vi "distancepidinit.vi"(10 "Distance From Target":dbl) -> (1 "Done?":bool)   [LabVIEW 2013]
uses:
  <vilib>/addons/control/pid/pid.llb/PID (DBL).vi
  <vilib>/Rock Robotics/WPI/RobotDrive/WPI_RobotDriveArcadeDrive_Standard(NoSaturation).vi
  <vilib>/Rock Robotics/WPI/RobotDrive/WPI_RobotDriveGetSetRefNum.vi
  <vilib>/addons/control/pid/NI_PID_pid.lvlib
panel:
  in  "reinitialize? (F)":bool
  in  "PID Gains Distance":T1={"proportional gain (Kc)"=0.3, "integral time (Ti, min)"=0.0, "derivative time (Td, min)"=0.0} {"derivative time (Td, min)" format="%.3f"; "integral time (Ti, min)" format="%.3f"; "proportional gain (Kc)" format="%.3f"}
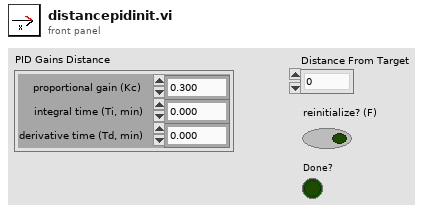
[diagram p1: front panel]
types:
  T1 = cluster{"proportional gain (Kc)":dbl, "integral time (Ti, min)":dbl, "derivative time (Td, min)":dbl}
  T2 = typedef "WPI_EncoderDevRef.ctl" = cluster{"DevStatus":errorcluster, "EncoderIndex":T3, "CounterIndex":T4, "DistancePerCount":dbl, "Decoding Type":T5}
  T3 = typedef "FPGA_EncoderIdx.ctl" = enum8{"Enc 0", "Enc 1", "Enc 2", "Enc 3", "Invalid"}
  T4 = typedef "FPGA_CounterCtrSystemIndex.ctl" = enum8{"Ctr 0", "Ctr 1", "Ctr 2", "Ctr 3", "Ctr 4", "Ctr 5", "Ctr 6", "Ctr 7", "Invalid"}
  T5 = typedef "WPI_EncoderType.ctl" = enum16{"1x", "2x", "4x"}
  T6 = typedef "WPI_RobotDriveDevRef.ctl" = cluster{"DevStatus":errorcluster, "Motors[]":T7[], "Square Inputs":bool, "Max Output":dbl, "Isochronous":bool}
  T7 = typedef "WPI_MotorControlDeviceRef.ctl" = cluster{"DeviceStatus":errorcluster, "Type":enum16{"PWM", "CAN"}, "PWM":cluster{"Digital Module":T8, "PWM Channel":T9, "DeadBand":T10}, "CAN":cluster{"Device Number":u8, "Control Mode":T11, "Semaphore":T12, "Max Vout":dbl}, "Invert":bool, "TransformRef":T13, "InvTransformRef":T13}
  T8 = typedef "FPGA_TypedefDigitalModule.ctl" = enum16{"Digital Module 1", "Digital Module 2"}
  T9 = typedef "FPGA_DIOPWMChannel.ctl" = enum8{"PWM 1", "PWM 2", "PWM 3", "PWM 4", "PWM 5", "PWM 6", "PWM 7", "PWM 8", "PWM 9", "PWM 10", "Invalid"}
  T10 = typedef "WPI_PWMDeadband.ctl" = cluster{"Name":string, "maxPositivePwm":i32, "minPositivePwm":i32, "centerPwm":i32, "maxNegativePwm":i32, "minNegativePwm":i32, "angularRange":u16}
  T11 = typedef "WPI_CANJaguar_ControlMode.ctl" = enum8{"Percent VBus", "Current", "Speed", "Position", "Voltage"}
  T12 = typedef "Semaphore RefNum" = refnum<k1>
  T13 = typedef "WPI_PWMTransform_ConPane.ctl" = refnum<vi>
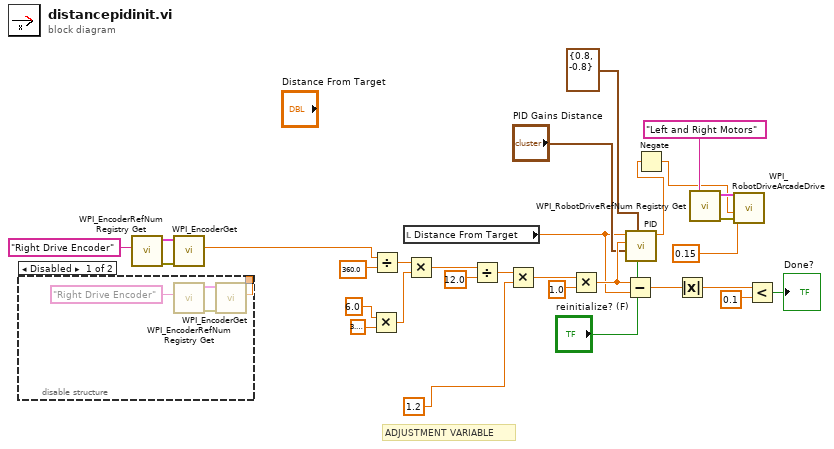
[diagram p0: block diagram]
diagram:
  # "ADJUSTMENT VARIABLE"
  n1 = disable-structure shown="Disabled" {
    disable-tunnel: [w34 _] -> _
    frame Disabled {
      n2 = call <vilib>:"WPI_EncoderRefNum Registry Get.vi"("refnum name"="Right Drive Encoder") -> ("error out"=w31:errorcluster, "EncoderDevRef"=w32:T2)  [unwired: 9 in]
      n3 = call <vilib>:"WPI_EncoderGet.vi"("error in (no error)"=w31, "EncoderDevRef"=w32) -> ("Distance"=w34:dbl)  [unwired: 4 in, 5 out]
    }
    frame Enabled {
    }
  }
  n4 = call <vilib>:"WPI_EncoderRefNum Registry Get.vi"("refnum name"="Right Drive Encoder") -> ("error out"=w18:errorcluster, "EncoderDevRef"=w19:T2)  [unwired: 9 in]
  n5 = call <vilib>:"WPI_EncoderGet.vi"("error in (no error)"=w18, "EncoderDevRef"=w19) -> ("Distance"=w2:dbl)  [unwired: 4 in, 5 out]
  n6 = Multiply(x=6.0, y=3.141592653589793) -> (x*y=w25:dbl)
  n7 = Divide(x=w2, y=360.0) -> (x/y=w24:dbl)
  n8 = local read "Distance From Target"() -> (w10:dbl)
  n9 = Multiply(x=w24, y=w25) -> (x*y=w26:dbl)
  n10 = Divide(x=w26, y=12.0) -> (x/y=w16:dbl)
  n11 = Multiply(x=w16, y=1.2) -> (x*y=w15:dbl)
  n12 = Multiply(x=w15, y=1.0) -> (x*y=w13:dbl)
  n13 = Subtract(x=w13, y=w10) -> (x-y=w28:dbl)
  n14 = call-poly <vilib>:"PID.vi"("reinitialize? (F)"="reinitialize? (F)", "output range"=cluster{"output high":dbl, "output low":dbl} {"output high"=0.8, "output low"=-0.8}, "PID gains"="PID Gains Distance", "process variable"=w13, "setpoint"=w10) -> ("output"=w3:dbl)  [unwired: 5 in, 1 out]
  n15 = Negate(x=w3) -> (-x=w4:dbl)
  n16 = Absolute Value(x=w28) -> (abs(x)=w29:dbl)
  n17 = call <vilib>:"WPI_RobotDriveRefNum Registry Get.vi"("refnum name"="Left and Right Motors") -> ("error out"=w8:errorcluster, "RobotDriveDevRef"=w7:T6)  [unwired: 9 in]
  n18 = call-poly <vilib>:"WPI_RobotDriveArcadeDrive.vi"("error in (no error)"=w8, "Y axis value"=w4, "X axis value"=0.15, "RobotDriveDevRef"=w7) -> ()  [unwired: 5 in, 3 out]
  n19 = Less?(x=w29, y=0.1) -> (x < y?=→"Done?":bool)
